vi "set_CW_laser.vi"() -> ()   [LabVIEW 2014]
panel:
  in  "Num Bytes to Fetch (64)":u8=64 min=1
  out "error out":errorcluster
  in  "Address (0x50)":u16=80 max=1023 format="%.0x"
  in  "Aardvark Handle":i32 min=0
  in  "error in (no error)":errorcluster
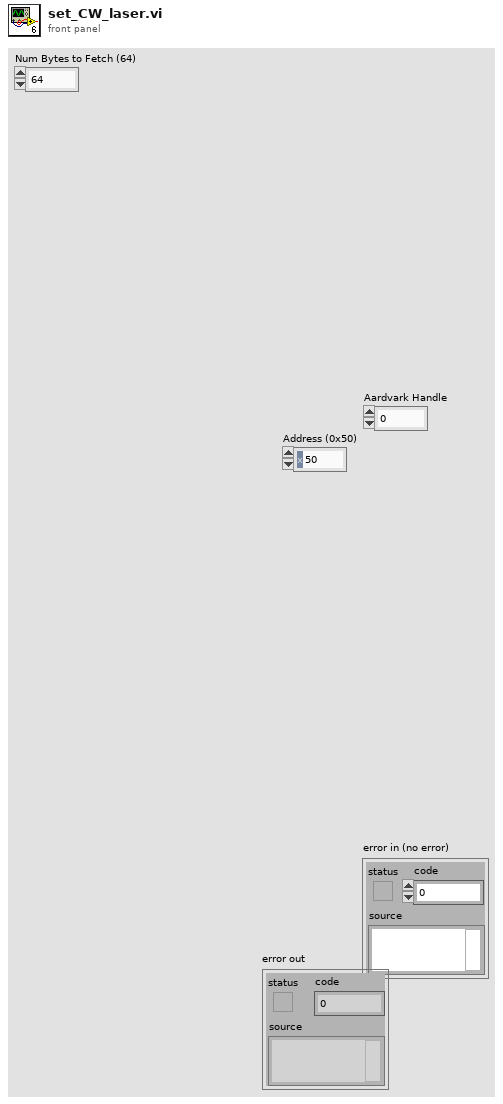
[diagram p1: front panel]
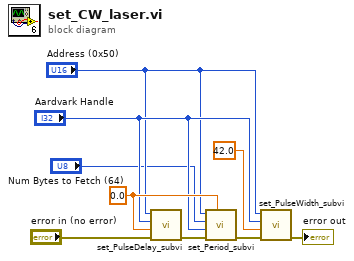
[diagram p0: block diagram]
diagram:
  w7 = 0.0
  n1 = call "set_PulseDelay_subvi.vi"("error in (no error)"="error in (no error)", "Pulse Delay"=w7, "Aardvark Handle"="Aardvark Handle", "Address (0x50) in"="Address (0x50)") -> ("error out"=w8:errorcluster)  [unwired: 7 in]
  n2 = call "set_Period_subvi.vi"("Period"=w7, "error in (no error)"=w8, "Aardvark Handle"="Aardvark Handle", "Num Bytes to Fetch (64) in"="Num Bytes to Fetch (64)", "Address (0x50) in"="Address (0x50)") -> ("error out"=w6:errorcluster)  [unwired: 6 in]
  n3 = call "set_PulseWidth_subvi.vi"("error in (no error)"=w6, "Pulsewidth"=42.0, "Aardvark Handle"="Aardvark Handle", "Address (0x50) in"="Address (0x50)") -> ("error out"=→"error out":errorcluster)  [unwired: 7 in]
